vi "PCO_GetFlimImageProcessingFlow.vi"(0 "ph":u64, 11 "error in (no error)":errorcluster {"code" format="%x"}) -> (3 "wOutputMode":u16(ring) items=["normal", "multiply x2"], 4 "ph out":u64, 6 "ErrorMessage":i32 format="%x", 8 "wAsymmetryCorrection":u16(ring) items=["OFF", "ON"], 15 "error out":errorcluster {"code" format="%x"})   [LabVIEW 2019, in "SDK.lvlib" / "SpecialCommandsFlim.lvlib"]
doc: "<b>Description:</b>\nGet settings of pco.flim specific internal image processing inside the camera.\n\n<b>Supported camera type:</b>\npco.flim\n\n<b>Descriptor dependency:</b>\nNone"
uses:
  SpecialCommandsFlim.lvlib
panel:
  out "wThresholdHigh":u16
  out "wThresholdLow":u16
  out "wReferencingMode":u16
  out "wCalculationMode":u16
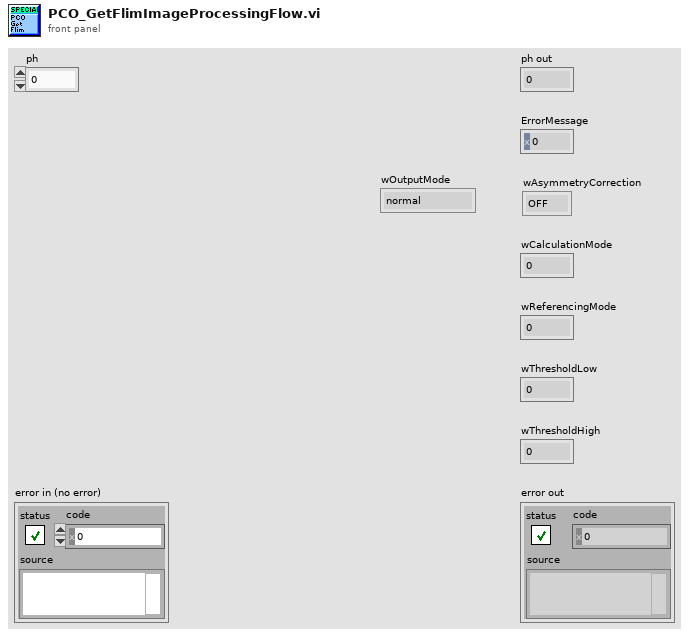
[diagram p1: front panel]
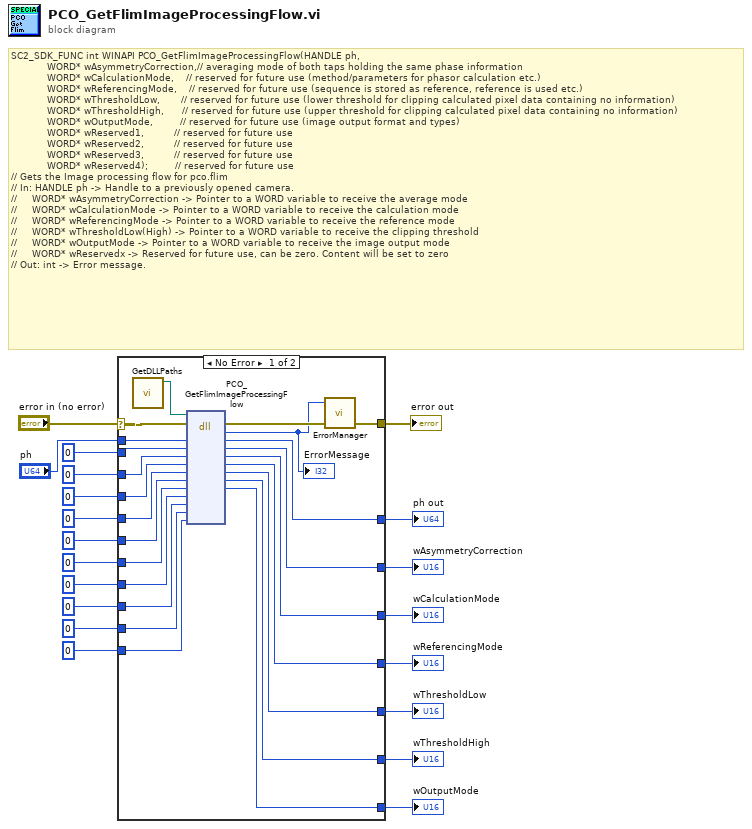
[diagram p0: block diagram]
diagram:
  # "SC2_SDK_FUNC int WINAPI PCO_GetFlimImageProcessingFlow(HANDLE ph, \n            WORD* wAsymmetryCorrection,// averaging mode of both taps holding the same phase information\n            WORD* wCalculationMode,    // reserved for future use (method/parameters for phasor calculation etc.)\n            WORD* wReferencingMode,    // reserved for future use (sequence is stored as reference, reference is used etc.)\n            WORD* wThresholdLow,       // reserved for future use (lower threshold for clipping calculated pixel data containing no information)\n            WORD* wThresholdHigh,      // reserved for future use (upper threshold for clipping calculated pixel data containing no information)\n            WORD* wOutputMode,         // reserved for future use (image output format and types)\n            WORD* wReserved1,          // reserved for future use\n            WORD* wReserved2,          // reserved for future use\n            WORD* wReserved3,          // reserved for future use\n            WORD* wReserved4);         // reserved for future use\n// Gets the Image processing flow for pco.flim\n// In: HANDLE ph -> Handle to a previously opened camera.\n//     WORD* wAsymmetryCorrection -> Pointer to a WORD variable to receive the average mode\n//     WORD* wCalculationMode -> Pointer to a WORD variable to receive the calculation mode\n//     WORD* wReferencingMode -> Pointer to a WORD variable to receive the reference mode\n//     WORD* wThresholdLow(High) -> Pointer to a WORD variable to receive the clipping threshold\n//     WORD* wOutputMode -> Pointer to a WORD variable to receive the image output mode\n//     WORD* wReservedx -> Reserved for future use, can be zero. Content will be set to zero\n// Out: int -> Error message."
  n1 = case shown="No Error" "error in (no error)" {
    selector: "error in (no error)" -> [w25 w51]
    tunnel: "ph" -> [w43 w50]
    tunnel: [w42 w50] -> w19
    tunnel: u16 0 ("wAsymmetryCorrection") -> [w41 w49]
    tunnel: [w40 w49] -> w17
    tunnel: u16 0 ("wCalculationMode") -> [w39 w48]
    tunnel: [w38 w48] -> w15
    tunnel: u16 0 ("wReferencingMode") -> [w37 w47]
    tunnel: [w36 w47] -> w13
    tunnel: u16 0 ("wThresholdLow") -> [w35 w46]
    tunnel: [w34 w46] -> w11
    tunnel: u16 0 ("wThresholdHigh") -> [w33 w45]
    tunnel: [w32 w45] -> w9
    tunnel: u16 0 ("wOutputMode") -> [w31 w44]
    tunnel: [w30 w44] -> w7
    tunnel: u16 0 ("wReserved1") -> [w29 _]
    tunnel: u16 0 ("wReserved2") -> [w28 _]
    tunnel: u16 0 ("wReserved3") -> [w27 _]
    tunnel: u16 0 ("wReserved4") -> [w26 _]
    tunnel: [w24 w51] -> w2
    frame No Error {
      n2 = call "GetDLLPaths.vi"() -> ("SC2_Cam_Path"=w21:path)  [unwired: 8 in, 3 out]
      n3 = dll-call lib="?" fn="PCO_GetFlimImageProcessingFlow"(path in=w21, error in=w25, "ph"=w43, "wAsymmetryCorrection"=w41, "wCalculationMode"=w39, "wReferencingMode"=w37, "wThresholdLow"=w35, "wThresholdHigh"=w33, "wOutputMode"=w31, "wReserved1"=w29, "wReserved2"=w28, "wReserved3"=w27, "wReserved4"=w26) -> (error out=w23:errorcluster, "return type"=w22:i32, "ph"=w42:u64, "wAsymmetryCorrection"=w40:u16, "wCalculationMode"=w38:u16, "wReferencingMode"=w36:u16, "wThresholdLow"=w34:u16, "wThresholdHigh"=w32:u16, "wOutputMode"=w30:u16)  [unwired: 5 in, 1 out]
      "ErrorMessage" <- w22
      n4 = call "ErrorManager.vi"("error in (no error)"=w23, "error code"=w22) -> ("error out"=w24:errorcluster)  [unwired: 2 in, 1 out]
    }
    frame Error {
    }
  }
  "ph out" <- w19
  "wAsymmetryCorrection" <- w17
  "wCalculationMode" <- w15
  "wReferencingMode" <- w13
  "wThresholdLow" <- w11
  "wThresholdHigh" <- w9
  "wOutputMode" <- w7
  "error out" <- w2
